vi "Read Gates (Fast).vi"(7 "Micropulse # In":i32, 8 "error in (no error)":errorcluster, 11 "Test No.":u32) -> (0 "error out":errorcluster, 1 "dt (us)":dbl, 2 "Gates":T1={"Display Gate"={"Start"=0.0, "Length"=100.0}, "ETM Mode"=enum."Echo Trigger OFF", "Echo Gate"={"Start (us)"=0.0, "Length (us)"=100.0, "Threshold"=10, "Colour"=0}, "Insp Gates"=[]} {"Insp Gates"."Max # Peaks" max=64000 step=100; "Insp Gates"."Threshold" min=10 max=4095 step=10; "Insp Gates"."Length (us)" min=0.0 max=96000.0 step=100.0; "Insp Gates"."Start (us)" min=0.0 max=64000.0 step=100.0; "Echo Gate"."Threshold" min=10 max=4095 step=10; "Echo Gate"."Length (us)" min=0.0 max=96000.0 step=100.0; "Echo Gate"."Start (us)" min=0.0 max=64000.0 step=100.0; "Display Gate"."Length" min=0.0 max=64000.0 step=1000.0; "Display Gate"."Start" min=0.0 max=64000.0 step=1000.0}, 5 "Micropulse # Out":i32)   [LabVIEW 2026, in "MicroPulse_Driver.lvlib"]
uses:
  MicroPulse_Driver.lvlib
  Datatypes/subdatatypes/MP - Registry Gates.ctl
  Datatypes/MP - display gate.ctl
  Datatypes/MP - echo gate mode.ctl
  Datatypes/MP - echo gate parameters.ctl
  Datatypes/MP - multigate inspection gate parameters.ctl
  Datatypes/MP - hysteresis level.ctl
  Datatypes/MP - multigate mode.ctl
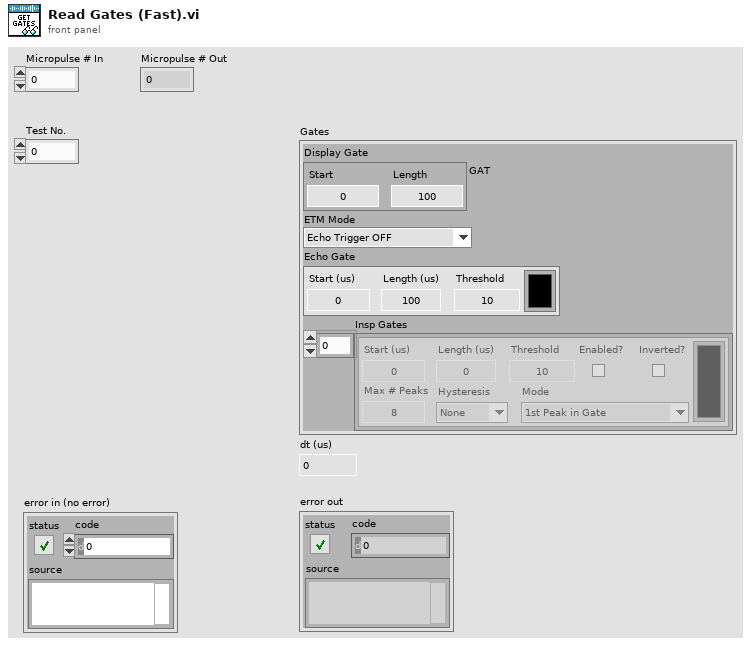
[diagram p1: front panel]
types:
  T1 = typedef "MicroPulse_Driver.lvlib/MP - Registry Gates.ctl" = cluster{"Display Gate":T2, "ETM Mode":T3, "Echo Gate":T4, "Insp Gates":T5[]}
  T2 = typedef "MicroPulse_Driver.lvlib/MP - display gate.ctl" = cluster{"Start":dbl, "Length":dbl}
  T3 = typedef "MicroPulse_Driver.lvlib/MP - echo gate mode.ctl" = enum16{"Echo Trigger OFF", "Echo Gate Display Mode", "Echo Trigger ON", "Multi Gate or FMC Mode", "Reserved", "PA - Echo Trigger ON"}
  T4 = typedef "MicroPulse_Driver.lvlib/MP - echo gate parameters.ctl" = cluster{"Start (us)":dbl, "Length (us)":dbl, "Threshold":u16, "Colour":u32}
  T5 = typedef "MicroPulse_Driver.lvlib/MP - multigate inspection gate parameters.ctl" = cluster{"Start (us)":dbl, "Length (us)":dbl, "Threshold":u16, "Enabled?":bool, "Max # Peaks":u16, "Hysteresis":T6, "Mode":T7, "Inverted?":bool, "Colour ":u32}
  T6 = typedef "MicroPulse_Driver.lvlib/MP - hysteresis level.ctl" = enum16{"None", "3dB", "6dB", "9dB", "12dB"}
  T7 = typedef "MicroPulse_Driver.lvlib/MP - multigate mode.ctl" = enum16{"1st Peak in Gate", "Largest Peak In Gate", "All Peaks In Gate", "1st Threshold Crossing"}
  T8 = typedef "MicroPulse_Driver.lvlib/MP-Registry Data-Cluster.ctl" = cluster{"Instrument Type":T9, "Serial #":u64, "Sample Frequency":T10, "dt (us)":dbl, "DOF":T11, "Material Velocity":dbl, "Asynch Reads":T12, "NUM of Tests":u32, "System Details":T13, "Gates":T1[], "Encoders":T15[], "CMD LUT":variant, "Command List":string}
  T9 = typedef "MicroPulse_Driver.lvlib/MP - instrument type.ctl" = enum16{"MicroPulse 5", "LT1", "LT2", "LTPA", "MPLT", "MicroPulse 6", "PipeScanner", "<MicroPulse>", "Micropulse 4", "Simulated Data"}
  T10 = typedef "MicroPulse_Driver.lvlib/MP - sample frequency.ctl" = enum16{"Use Default", "200MHz (LT2 only)", "100MHz", "50MHz", "25MHz", "10MHz"}
  T11 = typedef "MicroPulse_Driver.lvlib/MP - data output format.ctl" = enum16{"", "8-bit Mode", "10-bit Mode", "12-bit Mode", "16-bit Mode", "8-bit Log Mode", "12-bit Packed Mode"}
  T12 = typedef "MicroPulse_Driver.lvlib/MP - asynch read mode.ctl" = enum16{"Disabled", "Enabled"}
  T13 = typedef "MicroPulse_Driver.lvlib/MP - general system status.ctl" = cluster{"System Type":T9, "Serial No.":u64, "Channels":cluster{"Conv":u8, "PA":u16, "Extra":u32}, "Sample Frequency":cluster{"Default":u8, "Actual":u8}, "Software Versions":string, "Data Output Format":cluster{"Default":T11, "Actual":T11}, "Temperatures":cluster{"System":u8, "Processor":u8, "Slave Sys":u8, "Slave Proc":u8}, "Tx Buffer Size":u32, "System Error":string, "No. of Cards":u8, "DAC Gain":i16, "Uptimes":cluster{"since Power":u32, "since RSTS":u32, "since SRST":u32}, "Voltages":cluster{"Nominal":dbl, "Measured":dbl, "Difference":dbl}[], "Interface Cards":T14[]}
  T14 = typedef "MicroPulse_Driver.lvlib/MP - interface card status.ctl" = cluster{"Status":u8, "Map":u8, "Board - T":u8, "FPGA - T":u8, "PAIF Status":string, "Version":string}
  T15 = typedef "MicroPulse_Driver.lvlib/MP - encoder settings.ctl" = cluster{"Encoder Type":T16, "Counts/mm":u32, "Enable Termination?":bool, "Multiplier":u32, "Backlash Period (s)":dbl, "Encoder Filter":u32}
  T16 = typedef "MicroPulse_Driver.lvlib/MP - encoder type.ctl" = enum16{"Quadrature", "Step/Direction"}
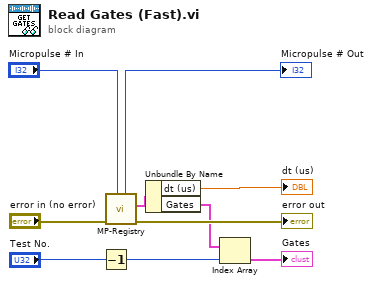
[diagram p0: block diagram]
diagram:
  n1 = Decrement(x="Test No.") -> (x-1=w1:u32)
  n2 = call "MP-Registry.vi"("Micropulse # In"="Micropulse # In", "error in (no error)"="error in (no error)") -> ("error out"=→"error out":errorcluster, "Micropulse Data"=w6:T8, "Micropulse # Out"=→"Micropulse # Out":i32)  [unwired: 6 in, 1 out]
  n3 = Unbundle By Name(w6) -> ("dt (us)"=→"dt (us)":dbl, "Gates"=w5:T1[])
  n4 = Index Array(array=w5, index=w1) -> (element=→"Gates":T1)
